vi "Documentation.vi"   [LabVIEW 2019, in "Inst.FP.lvclass"]
uses:
  Inst.FP.lvclass
  <userlib>/LevyLab/Instrument Framework/Instrument/API/Instrument.sendMessageToProcess (variant).vi
  <userlib>/LevyLab/Instrument Framework/Instrument/Instrument.lvclass
  <vilib>/JKI/JKI SMO/SMO/SMO.lvclass
  Typedefs/Inst.FP.Commands--Enum.ctl
  Typedefs/Inst.FP.getAll--Cluster.ctl
  Typedefs/Inst.FP.Configuration--Cluster.ctl
  Typedefs/Inst.FP.Type--Enum.ctl
  <userlib>/LevyLab/Instrument Framework/Instrument UI/Instrument UI.lvclass
  <vilib>/JKI/JKI SMO/SMO.UI/SMO.UI.lvclass
  <userlib>/LevyLab/RemoteControl/RemoteControl/RemoteControl.lvclass
  C:/Program Files (x86)/National Instruments/LabVIEW 2019/user.lib/LevyLab/Instrument Framework/Instrument Types/Cryostat/Instrument.Cryostat.lvclass
  C:/Program Files (x86)/National Instruments/LabVIEW 2019/user.lib/LevyLab/Instrument Framework/Instrument/Instrument.lvclass
  C:/Program Files (x86)/National Instruments/LabVIEW 2019/vi.lib/JKI/JKI SMO/SMO/SMO.lvclass
  C:/Program Files (x86)/National Instruments/LabVIEW 2019/vi.lib/JKI/JKI SMO/SMO.UI/SMO.UI.lvclass
types:
  T1 = typedef "Inst.FP.lvclass/Inst.FP.Configuration--Cluster.ctl" = cluster{"FP Type":T2, "Debug Mode":bool}
  T2 = typedef "Inst.FP.lvclass/Inst.FP.Type--Enum.ctl" = enum32{"Wet", "CF"}
  T3 = typedef "Inst.FP.lvclass/Inst.FP.getAll--Cluster.ctl" = cluster{"FP Data":dbl[], "MG Data":dbl[], "PT Data":dbl[], "Status Array":u32[], "Mode":string}
  T4 = typedef "Inst.FP.lvclass/Inst.FP.Commands--Enum.ctl" = enum16{"getMode", "setMode", "pushButton"}
  T5 = typedef "Instrument.lvlib/Instrument.lvclass/PublicEvents--Cluster.ctl" = cluster{"MessageFromProcess":refnum<user-event>}
  T6 = typedef "Instrument.lvlib/Instrument.lvclass/PrivateEvents--Cluster.ctl" = cluster{"MessageToProcess":refnum<user-event>, "LogData":refnum<user-event>, "LogDataMultiline":refnum<user-event>}
  T7 = typedef "Inst.FP.lvclass/PublicEvents--Cluster.ctl" = cluster{"MessageFromProcess":refnum<user-event>}
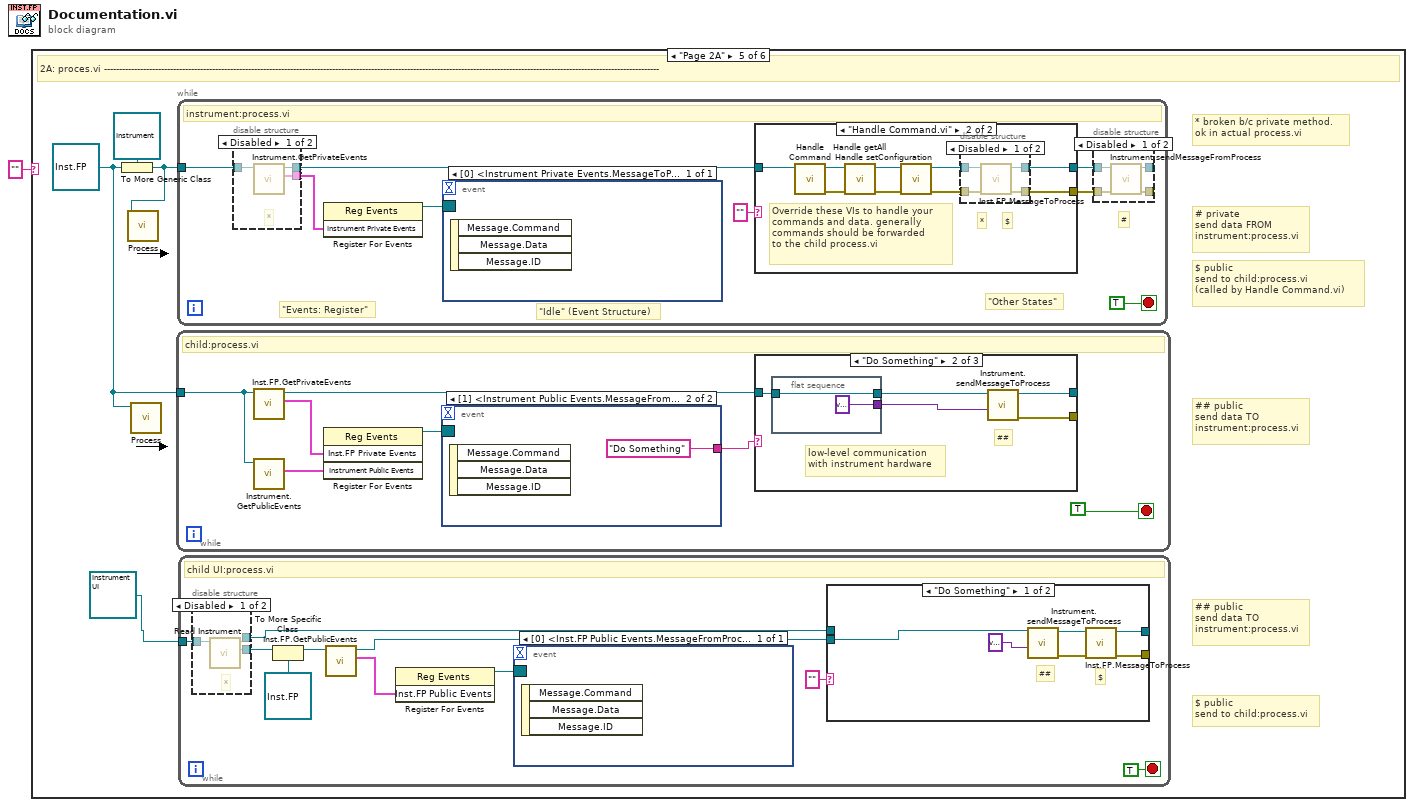
[diagram p0: block diagram]
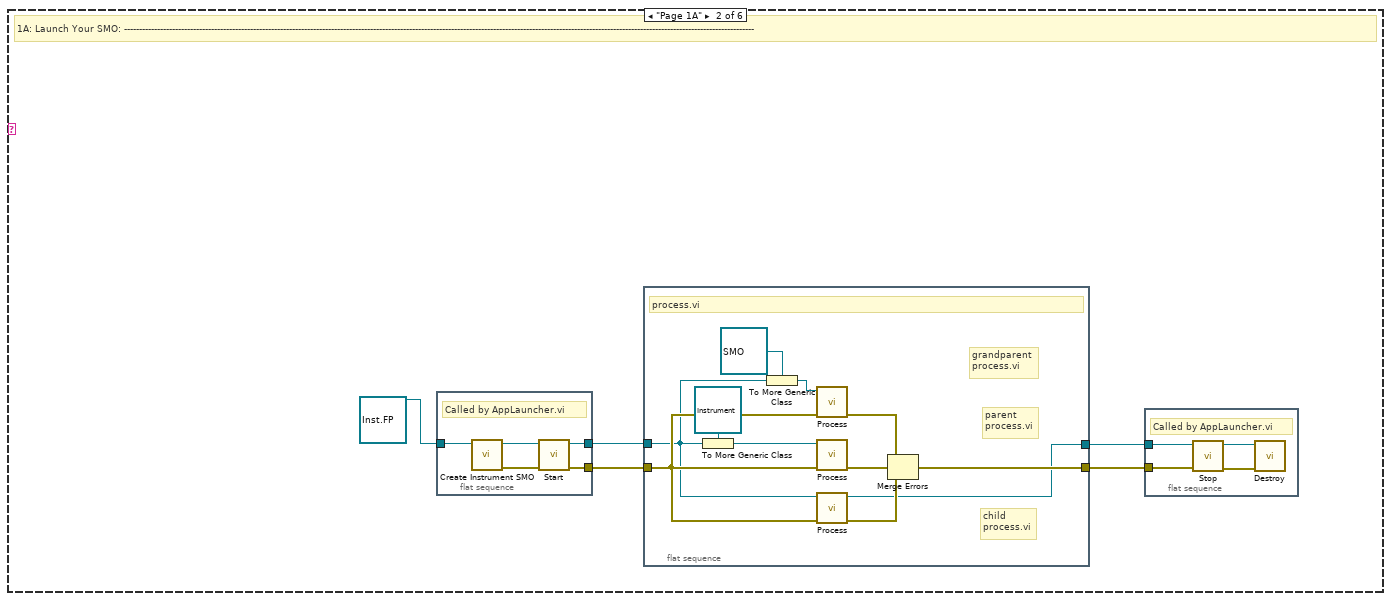
[diagram p3: hidden frame]
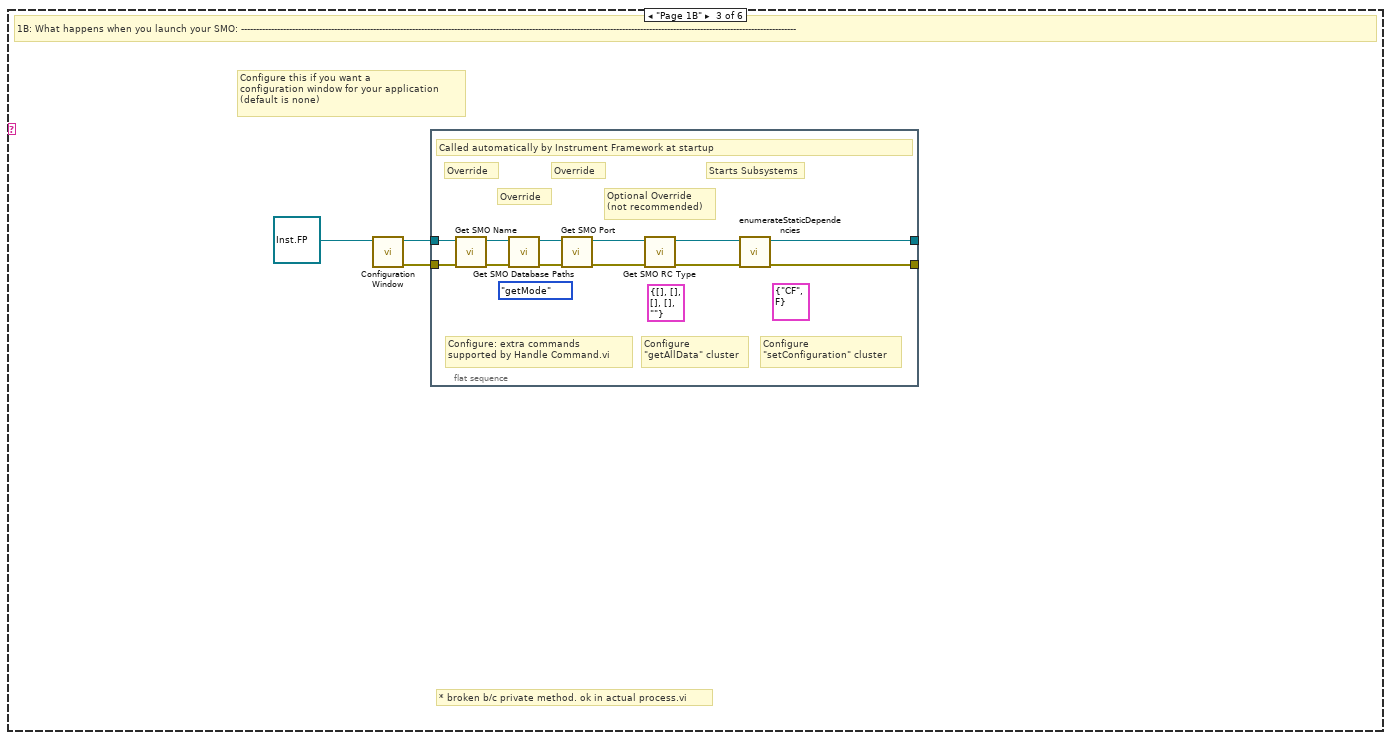
[diagram p4: hidden frame]
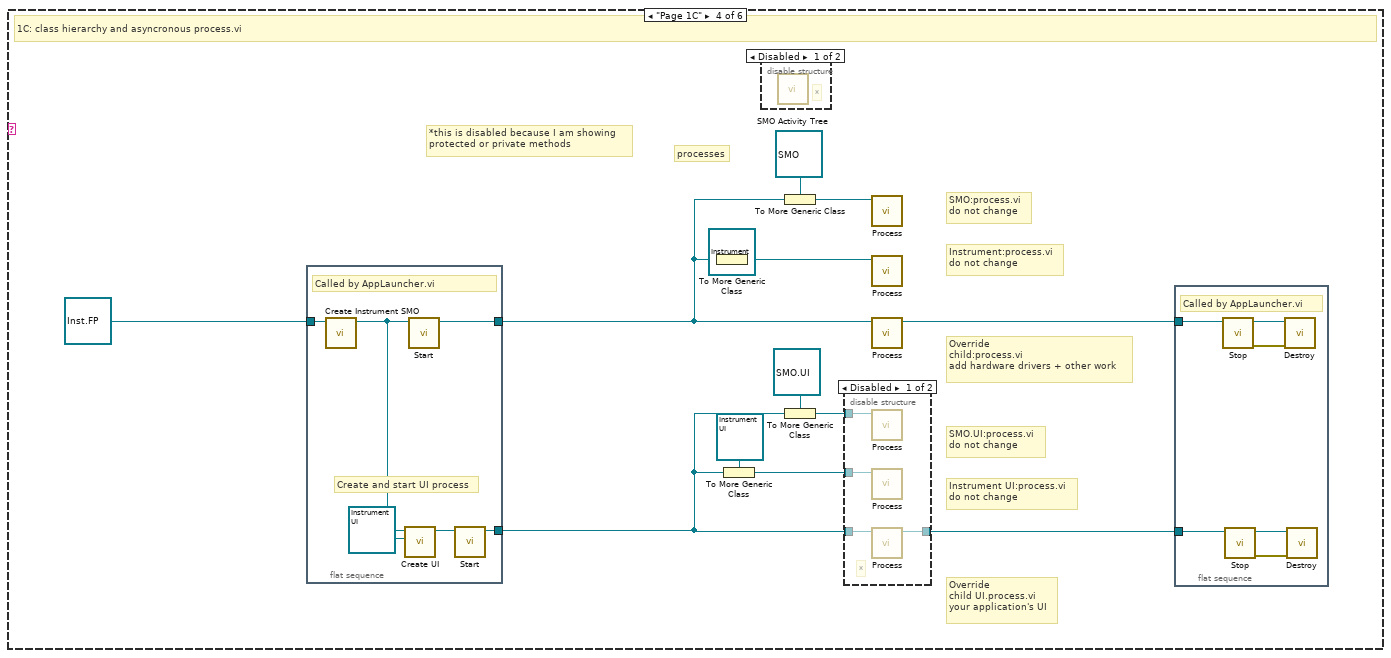
[diagram p5: hidden frame]
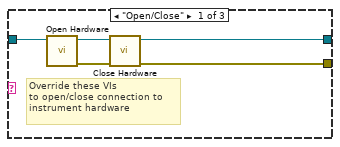
[diagram p10: hidden frame]
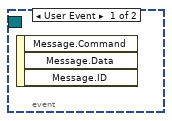
[diagram p12: hidden frame]
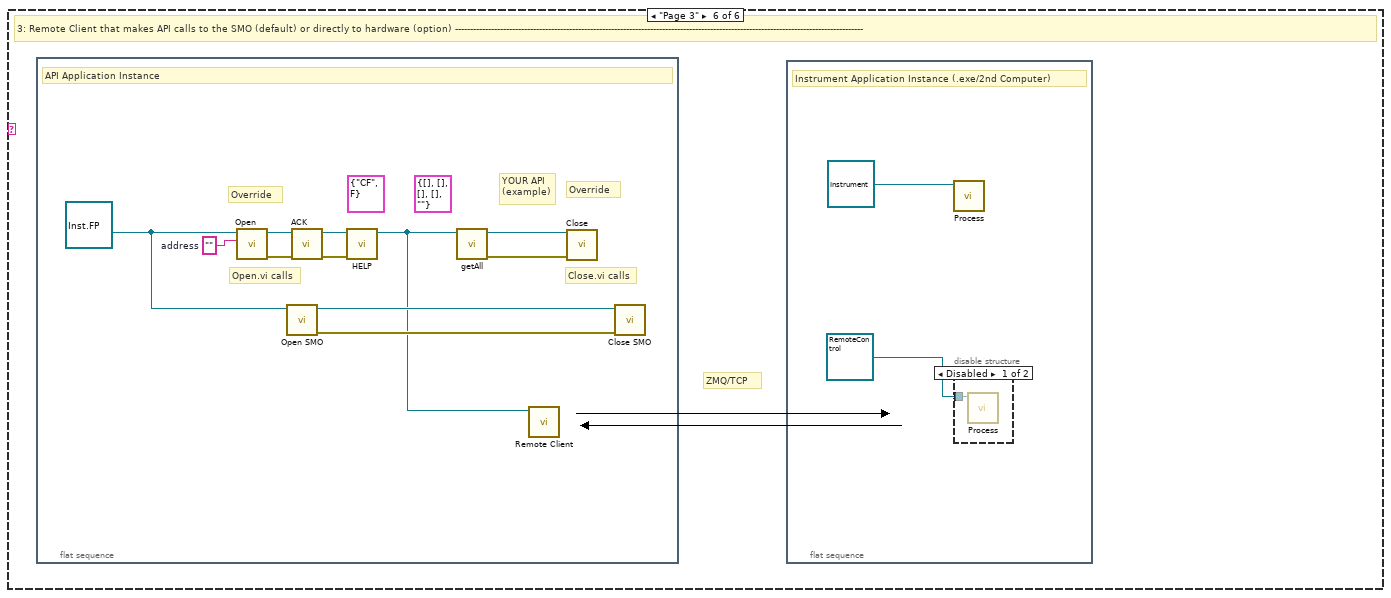
[diagram p17: hidden frame]
diagram:
  n1 = case shown="\"Page 2A\"" "" {
    frame Default {
    }
    frame "Page 1A" {
      # "1A: Launch Your SMO: ------------------------------------------------------------------------------------------------------------------------------------------------------------------------------------------------------------------"
      n2 = flat-sequence {
        tunnel: [w24] -> w3
        tunnel: [w23] -> w5
        tunnel: refnum<class "Inst.FP.lvclass"> refnum ("Instrument.Template.lvclass") -> [w22]
        frame #0 {
          # "Called by AppLauncher.vi"
          n3 = call <userlib>:"Create Instrument SMO.vi"("Instrument in"=w22) -> ("error out"=w25:errorcluster, "Instrument out"=w26:refnum<class "Inst.FP.lvclass">)  [unwired: 9 in]
          n4 = call <vilib>:"Start.vi"("error in (no error)"=w25, "SMO"=w26) -> ("error out"=w23:errorcluster, "SMO out"=w24:refnum<class "Inst.FP.lvclass">)  [unwired: 8 in]
        }
      }
      n5 = flat-sequence {
        tunnel: [w17] -> w6
        tunnel: w5 -> [w15]
        tunnel: [w9] -> w4
        tunnel: w3 -> [w8]
        frame #0 {
          # "child\nprocess.vi"
          # "grandparent\nprocess.vi"
          # "parent\nprocess.vi"
          # "process.vi"
          n6 = To More Generic Class(target class=refnum<class "Instrument.lvclass"> refnum ("Instrument"), reference=w8) -> (generic class reference=w14:refnum<class "Instrument.lvclass">)
          n7 = To More Generic Class(target class=refnum<class "SMO.lvclass"> refnum ("SMO"), reference=w8) -> (generic class reference=w16:refnum<class "SMO.lvclass">)
          n8 = call-dynamic "Process.vi"("error in"=w15, "SMO"=w16) -> ("error out"=w10:errorcluster)  [unwired: 8 in, 1 out]
          n9 = call-dynamic "Process.vi"("error in"=w15, "Instrument"=w14) -> ("error out"=w12:errorcluster)  [unwired: 8 in, 1 out]
          n10 = call-dynamic "Process.vi"("error in"=w15, "Inst.FP"=w8) -> ("error out"=w11:errorcluster, "Inst.FP out"=w9:refnum<class "Inst.FP.lvclass">)  [unwired: 8 in]
          n11 = Merge Errors(w10, w12, w11) -> (w17:errorcluster)
        }
      }
      n12 = flat-sequence {
        tunnel: w4 -> [w19]
        tunnel: w6 -> [w18]
        frame #0 {
          # "Called by AppLauncher.vi"
          n13 = call <vilib>:"Stop.vi"("error in (no error)"=w18, "SMO"=w19) -> ("error out"=w21:errorcluster, "SMO out"=w20:refnum<class "Inst.FP.lvclass">)  [unwired: 8 in]
          n14 = call <vilib>:"Destroy.vi"("error in (no error)"=w21, "SMO"=w20) -> ()  [unwired: 9 in, 1 out]
        }
      }
    }
    frame "Page 1B" {
      # "* broken b/c private method. ok in actual process.vi"
      # "Configure this if you want a\nconfiguration window for your application\n(default is none)"
      # "1B: What happens when you launch your SMO: -----------------------------------------------------------------------------------------------------------------------------------------------------------------------------------------"
      n15 = call-dynamic "Configuration Window.vi"("Inst.FP"=refnum<class "Inst.FP.lvclass"> refnum ("Instrument.Template.lvclass")) -> ("error out"=w28:errorcluster, "Inst.FP"=w29:refnum<class "Inst.FP.lvclass">)  [unwired: 9 in]
      n16 = flat-sequence {
        tunnel: w29 -> [w37]
        tunnel: w28 -> [w32]
        tunnel: [w31] -> _
        tunnel: [w30] -> _
        frame #0 {
          (unwired) T1 {"FP Type"=enum."CF", "Debug Mode"=FALSE} ("Configuration")
          (unwired) T3 {"FP Data"=[], "MG Data"=[], "PT Data"=[], "Status Array"=[], "Mode"=""} ("getAll")
          (unwired) Inst.FP.Commands--Enum."getMode" ("Commands")
          # "Configure\n\"setConfiguration\" cluster"
          # "Configure\n\"getAllData\" cluster"
          # "Configure: extra commands\nsupported by Handle Command.vi"
          # "Starts Subsystems"
          # "Override"
          # "Override"
          # "Override"
          # "Optional Override\n(not recommended)"
          # "Called automatically by Instrument Framework at startup"
          n17 = call-dynamic "Get SMO Name.vi"("error in (no error)"=w32, "Inst.FP in"=w37) -> ("error out"=w35:errorcluster, "Inst.FP out"=w36:refnum<class "Inst.FP.lvclass">)  [unwired: 7 in, 1 out]
          n18 = call-dynamic "Get SMO Database Paths.vi"("error in (no error)"=w35, "Inst.FP in"=w36) -> ("error out"=w33:errorcluster, "Inst.FP out"=w34:refnum<class "Inst.FP.lvclass">)  [unwired: 7 in, 1 out]
          n19 = call-dynamic "Get SMO Port.vi"("error in (no error)"=w33, "Inst.FPInstrument in"=w34) -> ("error out"=w38:errorcluster, "Inst.FPInstrument out"=w39:refnum<class "Inst.FP.lvclass">)  [unwired: 7 in, 1 out]
          n20 = call-dynamic "Get SMO RC Type.vi"("error in (no error)"=w38, "Instrument in"=w39) -> ("error out"=w40:errorcluster, "Instrument out"=w41:refnum<class "Inst.FP.lvclass">)  [unwired: 7 in, 1 out]
          n21 = call-dynamic "enumerateStaticDependencies.vi"("error in (no error)"=w40, "Instrument"=w41) -> ("error out"=w31:errorcluster, "Instrument out"=w30:refnum<class "Inst.FP.lvclass">)  [unwired: 7 in, 1 out]
        }
      }
    }
    frame "Page 1C" {
      # "processes"
      # "SMO.UI:process.vi\ndo not change"
      # "Instrument UI:process.vi\ndo not change"
      # "Override\nchild:process.vi\nadd hardware drivers + other work"
      # "SMO:process.vi\ndo not change"
      # "Instrument:process.vi\ndo not change"
      # "*this is disabled because I am showing\nprotected or private methods"
      # "Override\nchild UI.process.vi\nyour application's UI"
      # "1C: class hierarchy and asyncronous process.vi"
      n22 = flat-sequence {
        tunnel: [w70] -> w53
        tunnel: refnum<class "Inst.FP.lvclass"> refnum ("Instrument.Template.lvclass") -> [w69]
        tunnel: [w66] -> w52
        frame #0 {
          # "Create and start UI process"
          # "Called by AppLauncher.vi"
          n23 = call <userlib>:"Create Instrument SMO.vi"("Instrument in"=w69) -> ("Instrument out"=w68:refnum<class "Inst.FP.lvclass">)  [unwired: 9 in, 1 out]
          n24 = call <userlib>:"Create UI.vi"("Instrument in"=w68, "Instrument UI"=refnum<class "Instrument UI.lvclass"> refnum) -> ("Instrument UI out"=w67:refnum<class "Instrument UI.lvclass">)  [unwired: 8 in, 1 out]
          n25 = call <vilib>:"Start.vi"("SMO"=w68) -> ("SMO out"=w70:refnum<class "Inst.FP.lvclass">)  [unwired: 9 in, 1 out]
          n26 = call <vilib>:"Start.vi"("SMO"=w67) -> ("SMO out"=w66:refnum<class "Instrument UI.lvclass">)  [unwired: 9 in, 1 out]
        }
      }
      n27 = To More Generic Class(target class=refnum<class "Instrument.lvclass"> refnum ("Instrument"), reference=w53) -> (generic class reference=w49:refnum<class "Instrument.lvclass">)
      n28 = To More Generic Class(target class=refnum<class "Instrument UI.lvclass"> refnum ("Instrument UI"), reference=w52) -> (generic class reference=w45:refnum<class "Instrument UI.lvclass">)
      n29 = disable-structure shown="Disabled" {
        frame Disabled {
          # "*"
          n30 = call <vilib>:"SMO Activity Tree.vi"() -> ()  [unwired: 12 in]
        }
        frame Enabled {
        }
      }
      n31 = To More Generic Class(target class=refnum<class "SMO.lvclass"> refnum ("SMO"), reference=w53) -> (generic class reference=w50:refnum<class "SMO.lvclass">)
      n32 = To More Generic Class(target class=refnum<class "SMO.UI.lvclass"> refnum ("SMO.UI"), reference=w52) -> (generic class reference=w43:refnum<class "SMO.UI.lvclass">)
      n33 = disable-structure shown="Disabled" {
        disable-tunnel: w52 -> [w58 _]
        disable-tunnel: [w57 _] -> w51
        disable-tunnel: w45 -> [w56 _]
        disable-tunnel: w43 -> [w55 _]
        frame Disabled {
          # "*"
          n34 = call-dynamic "Process.vi"("SMO.UI"=w55) -> ()  [unwired: 9 in, 2 out]
          n35 = call-dynamic "Process.vi"("Instrument UI in"=w56) -> ()  [unwired: 9 in, 2 out]
          n36 = call-dynamic "Process.vi"("Instrument UI in"=w58) -> ("Instrument UI out"=w57:refnum<class "Instrument UI.lvclass">)  [unwired: 9 in, 1 out]
        }
        frame Enabled {
        }
      }
      n37 = call-dynamic "Process.vi"("SMO"=w50) -> ()  [unwired: 9 in, 2 out]
      n38 = call-dynamic "Process.vi"("Instrument"=w49) -> ()  [unwired: 9 in, 2 out]
      n39 = call-dynamic "Process.vi"("Inst.FP"=w53) -> ("Inst.FP out"=w54:refnum<class "Inst.FP.lvclass">)  [unwired: 9 in, 1 out]
      n40 = flat-sequence {
        tunnel: w54 -> [w62]
        tunnel: w51 -> [w60]
        frame #0 {
          # "Called by AppLauncher.vi"
          n41 = call <vilib>:"Stop.vi"("SMO"=w62) -> ("error out"=w64:errorcluster, "SMO out"=w63:refnum<class "Inst.FP.lvclass">)  [unwired: 9 in]
          n42 = call <vilib>:"Stop.vi"("SMO"=w60) -> ("error out"=w61:errorcluster, "SMO out"=w59:refnum<class "Instrument UI.lvclass">)  [unwired: 9 in]
          n43 = call <vilib>:"Destroy.vi"("error in (no error)"=w64, "SMO"=w63) -> ()  [unwired: 9 in, 1 out]
          n44 = call <vilib>:"Destroy.vi"("error in (no error)"=w61, "SMO"=w59) -> ()  [unwired: 9 in, 1 out]
        }
      }
    }
    frame "Page 2A" {
      w72 = refnum<class "Inst.FP.lvclass"> refnum ("Instrument.Template.lvclass")
      # "## public\nsend data TO\ninstrument:process.vi"
      # "$ public\nsend to child:process.vi"
      # "## public\nsend data TO\ninstrument:process.vi"
      # "$ public\nsend to child:process.vi\n(called by Handle Command.vi)"
      # "# private\nsend data FROM\ninstrument:process.vi"
      # "* broken b/c private method.\nok in actual process.vi"
      # "2A: proces.vi -----------------------------------------------------------------------------------------------------------------------------------------------------------------------------------------"
      n45 = To More Generic Class(target class=refnum<class "Instrument.lvclass"> refnum ("Instrument"), reference=w72) -> (generic class reference=w73:refnum<class "Instrument.lvclass">)
      n46 = call-dynamic "Process.vi"("Instrument"=w73) -> ()  [unwired: 9 in, 2 out]
      n47 = call-dynamic "Process.vi"("Inst.FP"=w72) -> ()  [unwired: 9 in, 2 out]
      n48 = while {
        tunnel: w72 -> [w98]
        stop <- TRUE stop-if-true
        # "child:process.vi"
        n49 = call "Inst.FP.GetPrivateEvents.vi"("Inst.FP in"=w98) -> ("Inst.FP Private Events"=w102:cluster{"MessageToProcess":refnum<user-event>}, "Inst.FP out"=w100:refnum<class "Inst.FP.lvclass">)  [unwired: 8 in, 1 out]
        n50 = call <userlib>:"Instrument.GetPublicEvents.vi"("Instrument"=w98) -> ("Instrument Public Events"=w99:T5)  [unwired: 8 in, 2 out]
        n51 = register-events(w102, w99) -> (reference out=w101:refnum<event-registration>)  [unwired: 2 in, 1 out]
        n52 = event shown="[1] <Instrument Public Events.MessageFromProcess>: User Event" {
          selector: w101 -> [_ _]
          dyn-events: _ -> [_ _]
          timeout: _ -> [_ _]
          tunnel: [_ "Do Something"] -> w96
          event User Event {
            n53 = event-data() -> ()  [unwired: 1 in, 3 out]
          }
          event User Event {
            n54 = event-data() -> ()  [unwired: 1 in, 3 out]
          }
        }
        n55 = case shown="\"Do Something\"" w96 {
          tunnel: w100 -> [w105 w110 w115]
          tunnel: [w104 w112 w115] -> _
          tunnel: [w103 w111 _] -> _
          frame "Open/Close" {
            # "Override these VIs\nto open/close connection to\ninstrument hardware"
            n56 = call-dynamic "Open Hardware.vi"("Instrument in"=w105) -> ("error out"=w107:errorcluster, "Instrument out"=w106:refnum<class "Inst.FP.lvclass">)  [unwired: 9 in]
            n57 = call-dynamic "Close Hardware.vi"("error in (no error)"=w107, "Instrument in"=w106) -> ("error out"=w103:errorcluster, "Instrument out"=w104:refnum<class "Inst.FP.lvclass">)  [unwired: 8 in]
          }
          frame "Do Something" {
            # "##"
            # "low-level communication\nwith instrument hardware"
            n58 = flat-sequence {
              tunnel: w110 -> [w114]
              tunnel: [w114] -> w109
              tunnel: [variant ("Data")] -> w108
              frame #0 {
              }
            }
            n59 = call-poly <userlib>:"Instrument.sendMessageToProcess.vi"("Data"=w108, "Instrument"=w109) -> ("error out"=w111:errorcluster, "Instrument out"=w112:refnum<class "Inst.FP.lvclass">)  [unwired: 8 in]
          }
          frame Default {
          }
        }
      }
      n60 = while {
        tunnel: w73 -> [w123]
        stop <- TRUE stop-if-true
        # "#"
        # "\"Other States\""
        # "\"Idle\" (Event Structure)"
        # "\"Events: Register\""
        # "instrument:process.vi"
        n61 = disable-structure shown="Disabled" {
          disable-tunnel: w123 -> [w147 w148]
          disable-tunnel: [w146 w148] -> w122
          disable-tunnel: [w145 _] -> w121
          frame Disabled {
            # "*"
            n62 = call <userlib>:"Instrument.GetPrivateEvents.vi"("Instrument"=w147) -> ("Instrument Private Events"=w145:T6, "Instrument out"=w146:refnum<class "Instrument.lvclass">)  [unwired: 8 in, 1 out]
          }
          frame Enabled {
          }
        }
        n63 = register-events(w121) -> (reference out=w120:refnum<event-registration>)  [unwired: 2 in, 1 out]
        n64 = event shown="[0] <Instrument Private Events.MessageToProcess>: User Event" {
          selector: w120 -> [_]
          dyn-events: _ -> [_]
          timeout: _ -> [_]
          event User Event {
            n65 = event-data() -> ()  [unwired: 1 in, 3 out]
          }
        }
        n66 = case shown="\"Handle Command.vi\"" "" {
          tunnel: w122 -> [w129 w138]
          tunnel: [w129 w132] -> w119
          tunnel: [_ w131] -> w118
          frame Default {
          }
          frame "Handle Command.vi" {
            # "*"
            # "$"
            # "Override these VIs to handle your\ncommands and data. generally \ncommands should be forwarded\nto the child process.vi"
            n67 = call-dynamic "Handle Command.vi"("Instrument in"=w138) -> ("error out"=w134:errorcluster, "Instrument out"=w137:refnum<class "Instrument.lvclass">)  [unwired: 7 in, 2 out]
            n68 = call-dynamic "Handle getAll.vi"("error in (no error)"=w134, "Instrument in"=w137) -> ("error out"=w135:errorcluster, "Instrument out"=w136:refnum<class "Instrument.lvclass">)  [unwired: 7 in, 1 out]
            n69 = call-dynamic "Handle setConfiguration.vi"("error in (no error)"=w135, "Instrument in"=w136) -> ("error out"=w130:errorcluster, "Instrument out"=w133:refnum<class "Instrument.lvclass">)  [unwired: 8 in]
            n70 = disable-structure shown="Disabled" {
              disable-tunnel: w133 -> [w139 w144]
              disable-tunnel: [w142 w144] -> w132
              disable-tunnel: [w141 w143] -> w131
              disable-tunnel: w130 -> [w140 w143]
              frame Disabled {
                n71 = call "Inst.FP.MessageToProcess.vi"("error in (no error)"=w140, "Inst.FP in"=w139) -> ("error out"=w141:errorcluster, "Inst.FP out"=w142:refnum<class "Inst.FP.lvclass">)  [unwired: 8 in]
              }
              frame Enabled {
              }
            }
          }
        }
        n72 = disable-structure shown="Disabled" {
          disable-tunnel: w119 -> [w125 _]
          disable-tunnel: w118 -> [w128 _]
          disable-tunnel: [w127 _] -> _
          disable-tunnel: [w126 _] -> _
          frame Disabled {
            n73 = call <userlib>:"Instrument.sendMessageFromProcess.vi"("error in (no error)"=w128, "Instrument"=w125) -> ("error out"=w127:errorcluster, "Instrument out"=w126:refnum<class "Instrument.lvclass">)  [unwired: 8 in]
          }
          frame Enabled {
          }
        }
      }
      n74 = while {
        tunnel: refnum<class "Instrument UI.lvclass"> refnum ("Instrument UI in") -> [w76]
        stop <- TRUE stop-if-true
        # "child UI:process.vi"
        n75 = disable-structure shown="Disabled" {
          disable-tunnel: [w94 _] -> w82
          disable-tunnel: [w92 w95] -> w75
          disable-tunnel: w76 -> [w93 w95]
          frame Disabled {
            # "*"
            n76 = call <userlib>:"Read Instrument.vi"("Instrument UI in"=w93) -> ("Instrument"=w94:refnum<class "Instrument.lvclass">, "Instrument UI"=w92:refnum<class "Instrument UI.lvclass">)  [unwired: 8 in, 1 out]
          }
          frame Enabled {
          }
        }
        n77 = To More Specific Class(target class=refnum<class "Inst.FP.lvclass"> refnum ("Instrument.Template.lvclass"), reference=w82) -> (specific class reference=w81:refnum<class "Inst.FP.lvclass">)  [unwired: 1 in, 1 out]
        n78 = call "Inst.FP.GetPublicEvents.vi"("Inst.FP in"=w81) -> ("Inst.FP Public Events"=w79:T7, "Inst.FP out"=w78:refnum<class "Inst.FP.lvclass">)  [unwired: 8 in, 1 out]
        n79 = register-events(w79) -> (reference out=w80:refnum<event-registration>)  [unwired: 2 in, 1 out]
        n80 = event shown="[0] <Inst.FP Public Events.MessageFromProcess>: User Event" {
          selector: w80 -> [_]
          dyn-events: _ -> [_]
          timeout: _ -> [_]
          event User Event {
            n81 = event-data() -> ()  [unwired: 1 in, 3 out]
          }
        }
        n82 = case shown="\"Do Something\"" "" {
          tunnel: w75 -> [_ _]
          tunnel: [w87 w91] -> _
          tunnel: [w86 _] -> _
          tunnel: w78 -> [w88 w91]
          frame "Do Something" {
            # "##"
            # "$"
            n83 = call-poly <userlib>:"Instrument.sendMessageToProcess.vi"("Data"=variant, "Instrument"=w88) -> ("error out"=w85:errorcluster, "Instrument out"=w89:refnum<class "Inst.FP.lvclass">)  [unwired: 8 in]
            n84 = call "Inst.FP.MessageToProcess.vi"("error in (no error)"=w85, "Inst.FP in"=w89) -> ("error out"=w86:errorcluster, "Inst.FP out"=w87:refnum<class "Inst.FP.lvclass">)  [unwired: 8 in]
          }
          frame Default {
          }
        }
      }
    }
    frame "Page 3" {
      # "ZMQ/TCP"
      # "3: Remote Client that makes API calls to the SMO (default) or directly to hardware (option) ----------------------------------------------------------------------------------------------------------------------------------------"
      n85 = flat-sequence {
        frame #0 {
          w157 = ""  # address
          (unwired) T1 {"FP Type"=enum."CF", "Debug Mode"=FALSE} ("Configuration")
          (unwired) T3 {"FP Data"=[], "MG Data"=[], "PT Data"=[], "Status Array"=[], "Mode"=""} ("getAll")
          w162 = refnum<class "Inst.FP.lvclass"> refnum ("Instrument.Template.lvclass")
          # "Close.vi calls"
          # "Open.vi calls"
          # "YOUR API\n(example)"
          # "Override"
          # "Override"
          # "API Application Instance"
          n86 = call-dynamic "Open.vi"("address"=w157, "Inst.FP in"=w162) -> ("error out"=w161:errorcluster, "Inst.FP out"=w160:refnum<class "Inst.FP.lvclass">)  [unwired: 8 in]
          n87 = call <userlib>:"Open SMO.vi"("Instrument in"=w162) -> ("error out"=w155:errorcluster, "Instrument out"=w156:refnum<class "Inst.FP.lvclass">)  [unwired: 9 in]
          n88 = call <userlib>:"ACK.vi"("error in (no error)"=w161, "Instrument in"=w160) -> ("error out"=w159:errorcluster, "Instrument out"=w158:refnum<class "Inst.FP.lvclass">)  [unwired: 7 in, 1 out]
          n89 = call <userlib>:"HELP.vi"("error in (no error)"=w159, "Instrument in"=w158) -> ("Instrument in"=w152:refnum<class "Inst.FP.lvclass">)  [unwired: 7 in, 2 out]
          n90 = call <userlib>:"getAll.vi"("Instrument in"=w152) -> ("error out"=w153:errorcluster, "Instrument out"=w154:refnum<class "Inst.FP.lvclass">)  [unwired: 8 in, 1 out]
          n91 = call <userlib>:"Remote Client.vi"("Instrument in"=w152) -> ()  [unwired: 7 in, 4 out]
          n92 = call-dynamic "Close.vi"("error in (no error)"=w153, "Inst.FP in"=w154) -> ()  [unwired: 8 in, 2 out]
          n93 = call <userlib>:"Close SMO.vi"("error in (no error)"=w155, "Instrument in"=w156) -> ()  [unwired: 8 in, 2 out]
        }
      }
      n94 = flat-sequence {
        frame #0 {
          # "Instrument Application Instance (.exe/2nd Computer)"
          n95 = call-dynamic "Process.vi"("Instrument"=refnum<class "Instrument.lvclass"> refnum) -> ()  [unwired: 9 in, 2 out]
          n96 = disable-structure shown="Disabled" {
            disable-tunnel: refnum<class "RemoteControl.lvclass"> refnum ("RemoteControl out") -> [w151 _]
            frame Disabled {
              n97 = call-dynamic "Process.vi"("RemoteControl"=w151) -> ()  [unwired: 9 in, 2 out]
            }
            frame Enabled {
            }
          }
        }
      }
    }
  }
